vi "Split String by Numbers.vi"(11 "String":string) -> (3 "Array":string[](array[string]))   [LabVIEW 2019, in "UI Common.lvlib"]
uses:
  UI Common.lvlib
  <vilib>/regexp/Match Regular Expression.xnode
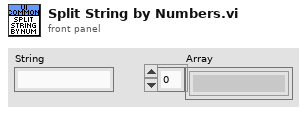
[diagram p1: front panel]
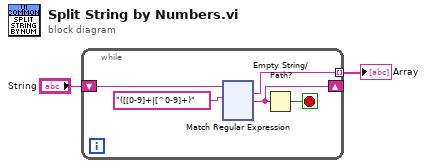
[diagram p0: block diagram]
diagram:
  n1 = while {
    shift-right: [w4] -> _
    shift-left: "String" -> [w6]
    tunnel: [w5] -> w2 mode=indexing
    stop <- w3 stop-if-true
    n2 = xnode "Match Regular Expression"("input string"=w6, "regular expression"="([[0-9]+|[^0-9]+)") -> ("whole match"=w5:string, "after match"=w4:string)  [unwired: 4 in, 3 out]
    n3 = Empty String/Path?(string/path=w4) -> (empty?=w3:bool)
  }
  "Array" <- w2
